vi "Wait till ready.vi"(8 "error in (no error)":errorcluster, 10 "Axis Number":i32, 11 ".NET Refnum in":T1) -> (0 "error out":errorcluster, 3 ".NET Refnum out":T1)   [LabVIEW 2016, in "Drivers.lvlib" / "Agilis.lvlib"]
uses:
  Agilis.lvlib
  AgilisCmdLib Refnum.ctl
  D:/Trace Grabber/Drivers/Agilis/AgilisCmdLib.dll
  AgilisCmdLib.dll
  Axis Status.ctl
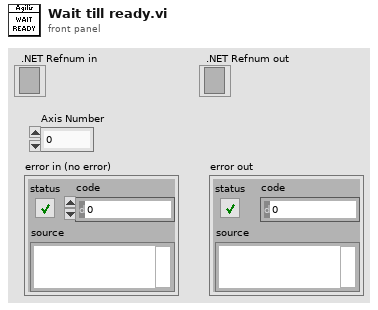
[diagram p1: front panel]
types:
  T1 = typedef "Drivers.lvlib/Agilis.lvlib/AgilisCmdLib Refnum.ctl" = refnum<k24>
  T2 = typedef "Drivers.lvlib/Agilis.lvlib/Axis Status.ctl" = i32
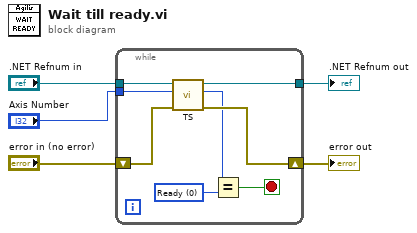
[diagram p0: block diagram]
diagram:
  n1 = while {
    tunnel: ".NET Refnum in" -> [w13]
    tunnel: [w11] -> w5
    shift-right: [w10] -> w2
    shift-left: "error in (no error)" -> [w12]
    tunnel: "Axis Number" -> [w9]
    stop <- w6 stop-if-true
    w7 = T2 0 items=["Ready", "Stepping", "Jogging", "Moving to limit"] ("y")
    n2 = call "TS.vi"("error in (no error)"=w12, "Axis Number"=w9, "Agilis in"=w13) -> ("error out"=w10:errorcluster, "Axis Status"=w8:T2, "Agilis out"=w11:T1)  [unwired: 6 in]
    n3 = Equal?(x=w8, y=w7) -> (x = y?=w6:bool)
  }
  "error out" <- w2
  ".NET Refnum out" <- w5
